vi "Autocomplete UI.vi"(0 "Allow Undefined Values? (F)":bool, 4 "LstBox Refnum":refnum<vi>, 5 "Ready Notifier":refnum<notifier>, 6 "Height (200)":i16=200, 7 "Stop Event":refnum<user-event>, 8 "Options":refnum<user-event>, 9 "Selection Event":refnum<user-event>, 10 "Autohide ListBox (F)":bool, 11 "Str Refnum":refnum<vi>) -> ()   [LabVIEW 2020, in "AutoComplete.lvlib"]
uses:
  AutoComplete.lvlib
  <vilib>/event_ctls.llb/eventvkey.ctl
panel:
  out "Revert":bool
  out "Starting Value":string
  in  "Visible":bool
  out "All Options":string[](array[string])
  in  "Listbox":i32(listbox)
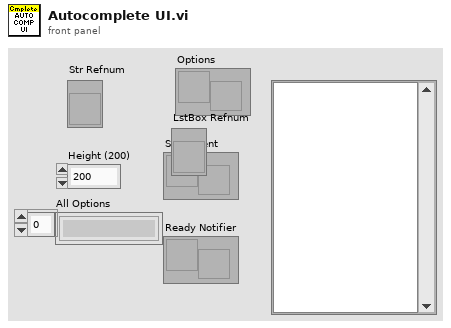
[diagram p1: front panel]
types:
  T1 = enum32{"Invalid", "Standard", "Closed", "Hidden", "Minimized", "Maximized"}
  T2 = typedef "eventvkey.ctl" = enum16{"ASCII", "Enter", "Return", "Shift", "Ctrl", "Alt", "Cmd", "Opt", "Caps", "NumLock", "Clear", "Break", "Up", "Down", "Left", "Right", "Insert", "Delete", "Home", "End", "PageUp", "PageDown", "Escape", "Help", "Pause", "ScrollLock", "F1", "F2", "F3", "F4", "F5", "F6", "F7", "F8", "F9", "F10", "F11", "F12", "F13", "F14", "F15", "F16", "F17", "F18", "F19", "F20", "F21", "F22", "F23", "F24", "Play", "VolumeUp", "VolumeDown", "Mute", "Two Byte Char"}
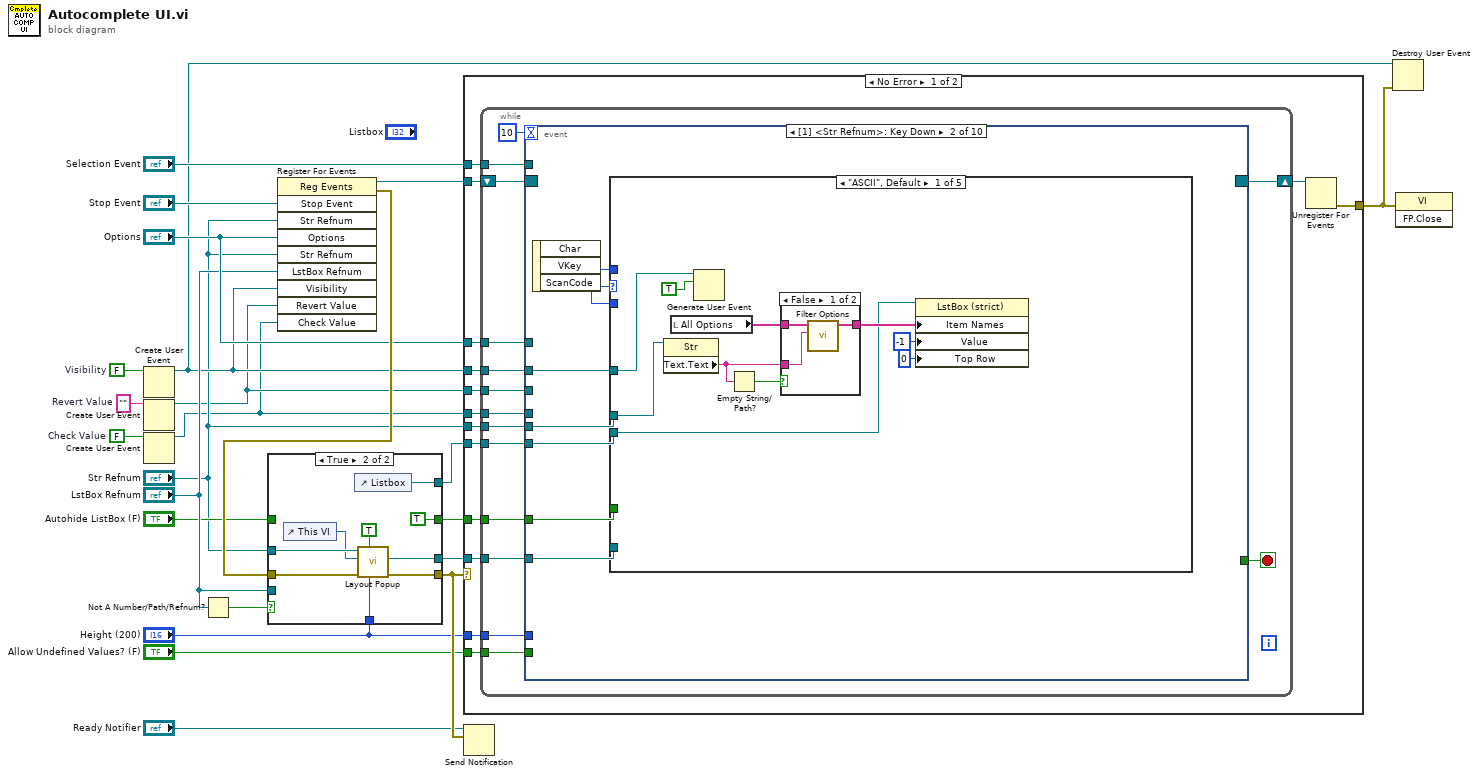
[diagram p0: block diagram]
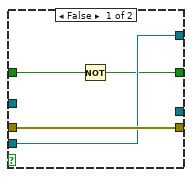
[diagram p2: hidden frame]
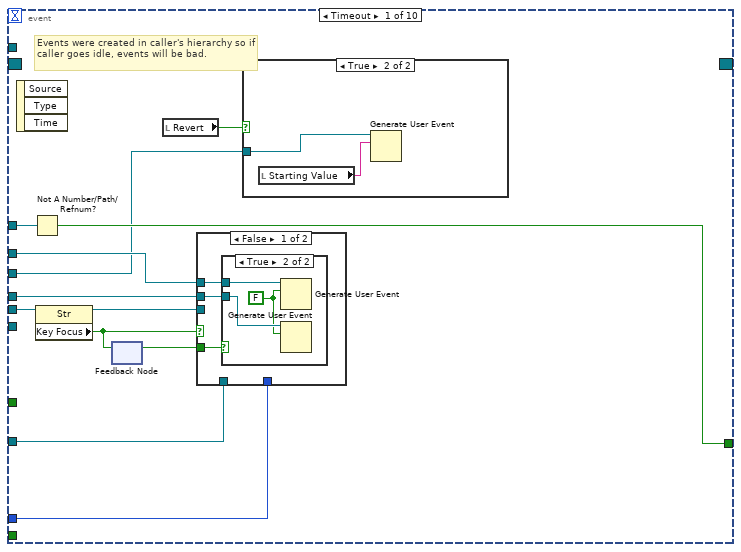
[diagram p3: hidden frame]
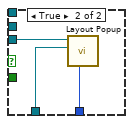
[diagram p6: hidden frame]
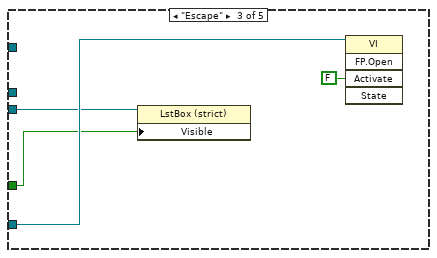
[diagram p9: hidden frame]
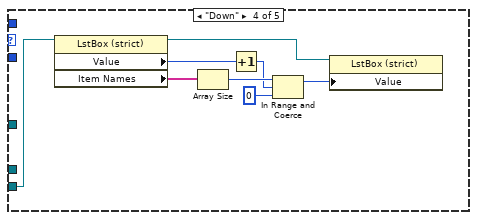
[diagram p10: hidden frame]
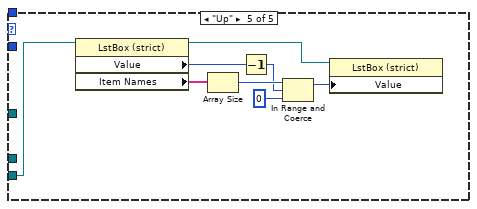
[diagram p11: hidden frame]
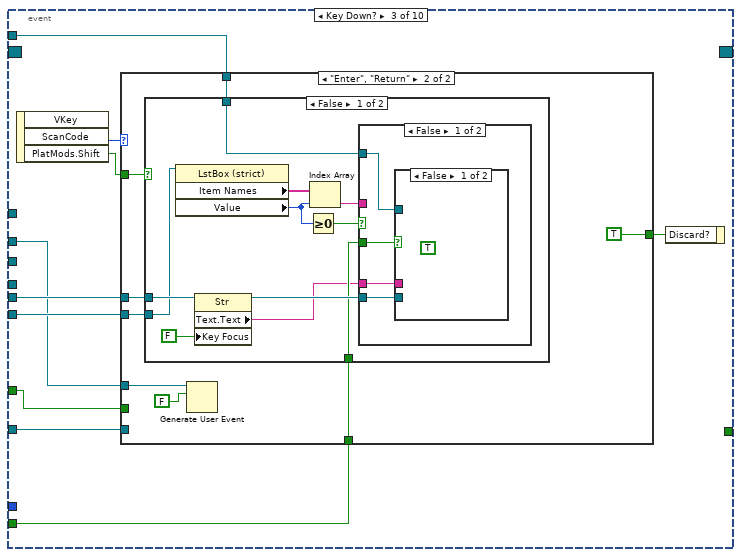
[diagram p12: hidden frame]
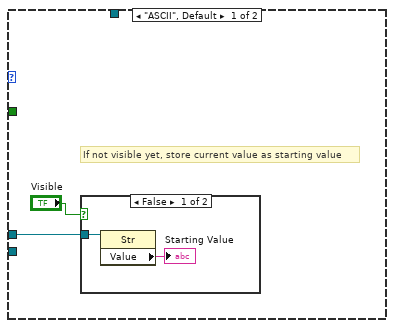
[diagram p13: hidden frame]
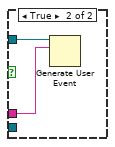
[diagram p15: hidden frame]
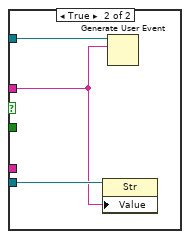
[diagram p16: hidden frame]
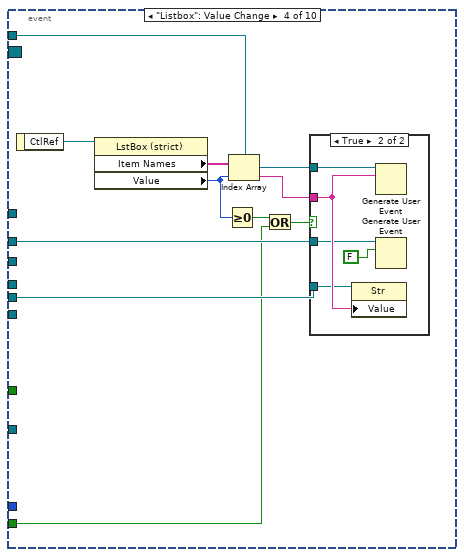
[diagram p18: hidden frame]
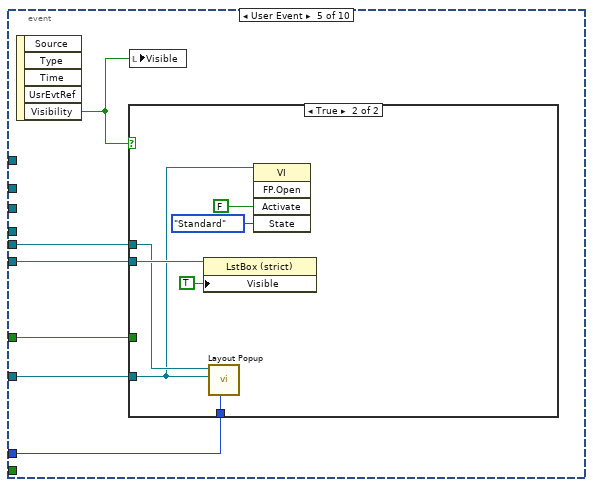
[diagram p20: hidden frame]
diagram:
  w2 = FALSE  # Check Value
  w4 = ""  # Revert Value
  w10 = FALSE  # Visibility
  n1 = Create User Event(user event datatype=w10) -> (user event=w8:refnum<user-event>)  [unwired: 1 in, 1 out]
  n2 = Create User Event(user event datatype=w4) -> (user event=w3:refnum<user-event>)  [unwired: 1 in, 1 out]
  n3 = Create User Event(user event datatype=w2) -> (user event=w1:refnum<user-event>)  [unwired: 1 in, 1 out]
  n4 = Not A Number/Path/Refnum?(number/path/refnum="LstBox Refnum") -> (NaN/Path/Refnum?=w16:bool)
  n5 = register-events("Stop Event", "Str Refnum", "Options", "Str Refnum", "LstBox Refnum", w8, w3, w1) -> (reference out=w21:refnum<event-registration>, error out=w22:errorcluster)  [unwired: 2 in]
  n6 = case shown="True" w16 {
    tunnel: w22 -> [w27 w30]
    tunnel: "Height (200)" -> [_ w32]
    tunnel: [_ w29] -> w20
    tunnel: [w27 w36] -> w23
    tunnel: "Str Refnum" -> [_ w33]
    tunnel: "LstBox Refnum" -> [w26 _]
    tunnel: [w26 w35] -> w15
    tunnel: [w24 TRUE] -> w14
    tunnel: "Autohide ListBox (F)" -> [w25 _]
    frame False {
      n7 = Not(x=w25) -> (.not. x?=w24:bool)
    }
    frame True {
      n8 = control-ref of="This VI"() -> (w31:refnum<vi>)
      n9 = control-ref of="Listbox"() -> (w35:refnum<vi>)
      n10 = call "Layout Popup.vi"("Height (200)"=w32, "Initial? (F)"=TRUE, "error in (no error)"=w30, "Popup VI In"=w31, "String Control In"=w33) -> ("error out"=w36:errorcluster, "Popup VI"=w29:refnum<vi>)  [unwired: 4 in, 1 out]
    }
  }
  n11 = case shown="No Error" w23 {
    tunnel: w21 -> [w50 _]
    tunnel: "Str Refnum" -> [w49 _]
    tunnel: [w47 _] -> w9
    tunnel: w20 -> [w46 _]
    tunnel: "Options" -> [w45 _]
    tunnel: w15 -> [w44 _]
    tunnel: w14 -> [w43 _]
    tunnel: "Selection Event" -> [w42 _]
    tunnel: w8 -> [w41 _]
    tunnel: "Height (200)" -> [w40 _]
    tunnel: "Allow Undefined Values? (F)" -> [w39 _]
    tunnel: w3 -> [w38 _]
    tunnel: w1 -> [w37 _]
    frame No Error {
      n12 = while {
        shift-right: [w64] -> w48
        shift-left: w50 -> [w65]
        tunnel: w49 -> [w62]
        tunnel: w46 -> [w60]
        tunnel: w45 -> [w59]
        tunnel: w44 -> [w58]
        tunnel: w43 -> [w57]
        tunnel: w42 -> [w56]
        tunnel: w41 -> [w55]
        tunnel: w40 -> [w54]
        tunnel: w39 -> [w53]
        tunnel: w38 -> [w52]
        tunnel: w37 -> [w51]
        stop <- w63 stop-if-true
        n13 = event shown="[1] <Str Refnum>: Key Down" {
          selector: w65 -> [_ _ _ _ _ _ _ _ _ _]
          dyn-events: [_ _ _ _ _ _ _ _ _ _] -> w64
          timeout: 10 -> [_ _ _ _ _ _ _ _ _ _]
          tunnel: [w75 _ _ _ _ TRUE _ _ _ _] -> w63
          tunnel: w62 -> [w77 w95 w137 w178 w190 _ w217 w221 w232 _]
          tunnel: w60 -> [w71 w92 w136 _ w193 _ _ _ _ _]
          tunnel: w59 -> [w76 _ _ _ _ w208 _ _ _ _]
          tunnel: w58 -> [_ w91 w135 _ w192 w211 w216 _ w231 _]
          tunnel: w57 -> [_ w90 w134 _ w191 w210 _ _ _ _]
          tunnel: w56 -> [_ _ w133 w177 _ w207 _ _ w230 _]
          tunnel: w55 -> [w74 w89 w132 w175 _ w209 _ _ _ _]
          tunnel: w54 -> [w70 _ _ _ w189 _ _ _ _ _]
          tunnel: w53 -> [_ _ w131 w173 _ _ _ _ w229 _]
          tunnel: w52 -> [w69 _ _ _ _ w206 _ _ _ _]
          tunnel: w51 -> [w66 _ _ _ _ _ _ _ _ _]
          event Timeout {
            # "Events were created in caller's hierarchy so if caller goes idle, events will be bad."
            n14 = event-data() -> ()  [unwired: 1 in, 3 out]
            n15 = Not A Number/Path/Refnum?(number/path/refnum=w76) -> (NaN/Path/Refnum?=w75:bool)
            n16 = property class="Str"(reference=w77) -> (reference out=w67:refnum<vi>, "Key Focus"=w73:bool)  [unwired: 1 in, 1 out]
            n17 = feedback-in #1(w73) -> ()
            n18 = feedback #1() -> (w72:bool)  [unwired: 1 in]
            n19 = local read "Revert"() -> (w68:bool)
            n20 = case shown="False" w73 {
              tunnel: w74 -> [w82 _]
              tunnel: w72 -> [w81 _]
              tunnel: w67 -> [_ w88]
              tunnel: w71 -> [_ w87]
              tunnel: w70 -> [_ w86]
              tunnel: w66 -> [w80 _]
              frame False {
                n21 = case shown="True" w81 {
                  tunnel: w82 -> [_ w85]
                  tunnel: w80 -> [_ w84]
                  frame False {
                  }
                  frame True {
                    w83 = FALSE ("event data")
                    n22 = Generate User Event(user event=w85, event data cluster=w83) -> ()  [unwired: 2 in, 2 out]
                    n23 = Generate User Event(user event=w84, event data cluster=w83) -> ()  [unwired: 2 in, 2 out]
                  }
                }
              }
              frame True {
                n24 = call "Layout Popup.vi"("Height (200)"=w86, "Popup VI In"=w87, "String Control In"=w88) -> ()  [unwired: 6 in, 3 out]
              }
            }
            n25 = case shown="True" w68 {
              tunnel: w69 -> [_ w79]
              frame False {
              }
              frame True {
                n26 = local read "Starting Value"() -> (w78:string)
                n27 = Generate User Event(user event=w79, event data cluster=w78) -> ()  [unwired: 2 in, 2 out]
              }
            }
          }
          event Key Down {
            n28 = event-data() -> ("Char"=w94:i16, "VKey"=w96:T2, "ScanCode"=w93:i16)  [unwired: 1 in]
            n29 = case shown="\"ASCII\", Default" w96 {
              tunnel: w95 -> [w105 _ _ _ _]
              tunnel: w94 -> [_ _ _ _ _]
              tunnel: w93 -> [_ _ _ _ _]
              tunnel: w92 -> [_ _ w113 _ _]
              tunnel: w91 -> [w99 _ w112 w116 w123]
              tunnel: w90 -> [_ _ w111 _ _]
              tunnel: w89 -> [w98 _ _ _ _]
              frame "ASCII", Default {
                n30 = property class="Str"(reference=w105) -> ("Text.Text"=w101:string)  [unwired: 1 in, 2 out]
                n31 = local read "All Options"() -> (w102:string[])
                n32 = Generate User Event(user event=w98, event data cluster=TRUE ("event data")) -> ()  [unwired: 2 in, 2 out]
                n33 = Empty String/Path?(string/path=w101) -> (empty?=w100:bool)
                n34 = case shown="False" w100 {
                  tunnel: [w107 w110] -> w103
                  tunnel: w102 -> [w109 w110]
                  tunnel: w101 -> [w108 _]
                  frame False {
                    n35 = call "Filter Options.vi"("Text"=w108, "All Options"=w109) -> ("Filtered Names"=w107:string[])  [unwired: 9 in]
                  }
                  frame True {
                  }
                }
                n36 = property on="Property Node" class="LstBox (strict)"(reference=w99, "Item Names"=w103, "Value"=-1 ("Listbox"), "Top Row"=0) -> ()  [unwired: 1 in, 2 out]
              }
              frame "Enter", "Return" {
                # "Handled in Key Down?"
              }
              frame "Escape" {
                n37 = property class="LstBox (strict)"(reference=w112, "Visible"=w111) -> ()  [unwired: 1 in, 2 out]
                n38 = invoke class="VI" method="FP.Open"(reference=w113, "Activate"=FALSE ("Activate?")) -> ()  [unwired: 3 in, 5 out]
              }
              frame "Down" {
                n39 = property on="Property Node" class="LstBox (strict)"(reference=w116) -> (reference out=w115:refnum<vi>, "Value"=w121:i32, "Item Names"=w122:string[])  [unwired: 1 in, 1 out]
                n40 = Array Size(array=w122) -> (size(s)=w120:i32)
                n41 = Increment(x=w121) -> (x+1=w119:i32)
                n42 = In Range and Coerce(upper limit=w120, x=w119, lower limit=0) -> (coerced(x)=w117:i32)  [unwired: 1 out]
                n43 = property on="Property Node" class="LstBox (strict)"(reference=w115, "Value"=w117) -> ()  [unwired: 1 in, 2 out]
              }
              frame "Up" {
                n44 = property on="Property Node" class="LstBox (strict)"(reference=w123) -> (reference out=w124:refnum<vi>, "Value"=w129:i32, "Item Names"=w130:string[])  [unwired: 1 in, 1 out]
                n45 = Array Size(array=w130) -> (size(s)=w128:i32)
                n46 = Decrement(x=w129) -> (x-1=w127:i32)
                n47 = In Range and Coerce(upper limit=w128, x=w127, lower limit=0) -> (coerced(x)=w125:i32)  [unwired: 1 out]
                n48 = property on="Property Node" class="LstBox (strict)"(reference=w124, "Value"=w125) -> ()  [unwired: 1 in, 2 out]
              }
            }
          }
          event Key Down? {
            n49 = event-data() -> ("VKey"=w140:T2, "PlatMods.Shift"=w139:bool)  [unwired: 1 in, 1 out]
            n50 = case shown="\"Enter\", \"Return\"" w140 {
              tunnel: w139 -> [_ w152]
              tunnel: [_ TRUE] -> w138
              tunnel: w137 -> [w142 w150]
              tunnel: w136 -> [_ _]
              tunnel: w135 -> [_ w149]
              tunnel: w134 -> [_ _]
              tunnel: w133 -> [_ w148]
              tunnel: w132 -> [_ w147]
              tunnel: w131 -> [_ w145]
              frame "ASCII", Default {
                # "If not visible yet, store current value as starting value"
                n51 = case shown="False" "Visible" {
                  tunnel: w142 -> [w144 _]
                  frame False {
                    n52 = property class="Str"(reference=w144) -> ("Value"=→"Starting Value":string)  [unwired: 1 in, 2 out]
                  }
                  frame True {
                  }
                }
              }
              frame "Enter", "Return" {
                n53 = case shown="False" w152 {
                  tunnel: w150 -> [w159 _]
                  tunnel: w149 -> [w157 _]
                  tunnel: w148 -> [w156 _]
                  tunnel: w145 -> [w154 _]
                  frame False {
                    n54 = property on="Property Node" class="LstBox (strict)"(reference=w157) -> ("Item Names"=w163:string[], "Value"=w162:i32)  [unwired: 1 in, 2 out]
                    n55 = property class="Str"(reference=w159, "Key Focus"=FALSE) -> (reference out=w158:refnum<vi>, "Text.Text"=w153:string)  [unwired: 1 in, 1 out]
                    n56 = Greater Or Equal To 0?(x=w162) -> (x >= 0?=w155:bool)
                    n57 = Index Array(array=w163, index=w162) -> (element=w161:string)
                    n58 = case shown="False" w155 {
                      tunnel: w161 -> [_ w170]
                      tunnel: w158 -> [w164 w172]
                      tunnel: w156 -> [w165 w171]
                      tunnel: w154 -> [w166 _]
                      tunnel: w153 -> [w167 _]
                      frame False {
                        n59 = case shown="False" w166 {
                          tunnel: w167 -> [_ w168]
                          tunnel: w165 -> [_ w169]
                          tunnel: w164 -> [_ _]
                          frame False {
                            (unwired) TRUE ("Revert")
                          }
                          frame True {
                            n60 = Generate User Event(user event=w169, event data cluster=w168) -> ()  [unwired: 2 in, 2 out]
                          }
                        }
                      }
                      frame True {
                        n61 = property class="Str"(reference=w172, "Value"=w170) -> ()  [unwired: 1 in, 2 out]
                        n62 = Generate User Event(user event=w171, event data cluster=w170) -> ()  [unwired: 2 in, 2 out]
                      }
                    }
                  }
                  frame True {
                  }
                }
                n63 = Generate User Event(user event=w147, event data cluster=FALSE ("event data")) -> ()  [unwired: 2 in, 2 out]
              }
            }
            n64 = event-data("Discard?"=w138) -> ()  [unwired: 1 in, 1 out]
          }
          event "Listbox": Value Change {
            n65 = event-data() -> ("CtlRef"=w176:refnum<vi>)  [unwired: 1 in]
            n66 = property on="Property Node" class="LstBox (strict)"(reference=w176) -> ("Item Names"=w182:string[], "Value"=w181:i32)  [unwired: 1 in, 2 out]
            n67 = Greater Or Equal To 0?(x=w181) -> (x >= 0?=w180:bool)
            n68 = Index Array(array=w182, index=w181) -> (element=w179:string)
            n69 = Or(x=w180, y=w173) -> (x .or. y?=w174:bool)
            n70 = case shown="True" w174 {
              tunnel: w179 -> [_ w187]
              tunnel: w178 -> [_ w186]
              tunnel: w177 -> [_ w185]
              tunnel: w175 -> [_ w184]
              frame False {
              }
              frame True {
                n71 = property class="Str"(reference=w186, "Value"=w187) -> ()  [unwired: 1 in, 2 out]
                n72 = Generate User Event(user event=w185, event data cluster=w187) -> ()  [unwired: 2 in, 2 out]
                n73 = Generate User Event(user event=w184, event data cluster=FALSE ("event data")) -> ()  [unwired: 2 in, 2 out]
              }
            }
          }
          event User Event {
            n74 = event-data() -> ("Visibility"=w188:bool)  [unwired: 1 in, 4 out]
            n75 = case shown="True" w188 {
              tunnel: w193 -> [w195 w200]
              tunnel: w192 -> [w197 w204]
              tunnel: w191 -> [w194 _]
              tunnel: w190 -> [_ w201]
              tunnel: w189 -> [_ w202]
              frame False {
                (unwired) FALSE
                n76 = property class="LstBox (strict)"(reference=w197, "Visible"=w194) -> ()  [unwired: 1 in, 2 out]
                n77 = invoke class="VI" method="FP.Open"(reference=w195, "Activate"=FALSE ("Activate?"), "State"=T1."Hidden") -> ()  [unwired: 2 in, 5 out]
              }
              frame True {
                n78 = property class="LstBox (strict)"(reference=w204, "Visible"=TRUE) -> ()  [unwired: 1 in, 2 out]
                n79 = call "Layout Popup.vi"("Height (200)"=w202, "Popup VI In"=w200, "String Control In"=w201) -> ()  [unwired: 6 in, 3 out]
                n80 = invoke class="VI" method="FP.Open"(reference=w200, "Activate"=FALSE ("Activate?"), "State"=T1."Standard") -> ()  [unwired: 2 in, 5 out]
              }
            }
            n81 = local write "Visible"(w188) -> ()
          }
          event User Event {
            n82 = event-data() -> ()  [unwired: 1 in, 1 out]
            n83 = Destroy User Event(user event=w207) -> ()  [unwired: 1 in, 1 out]
            n84 = Destroy User Event(user event=w206) -> ()  [unwired: 1 in, 1 out]
            n85 = Destroy User Event(user event=w209) -> ()  [unwired: 1 in, 1 out]
            n86 = property class="LstBox (strict)"(reference=w211, "Visible"=w210) -> ()  [unwired: 1 in, 2 out]
            n87 = Destroy User Event(user event=w208) -> ()  [unwired: 1 in, 1 out]
          }
          event User Event {
            # "Use this hidden indicator to store the full list of options since we'll be filtering down the displayed listbox."
            n88 = event-data() -> ("Options"=w215:string[])  [unwired: 1 in]
            "All Options" <- w215
            n89 = property class="Str"(reference=w217) -> ("Text.Text"=w214:string)  [unwired: 1 in, 2 out]
            n90 = call "Filter Options.vi"("Text"=w214, "All Options"=w215) -> ("Filtered Names"=w213:string[])  [unwired: 9 in]
            n91 = property on="Property Node" class="LstBox (strict)"(reference=w216, "Item Names"=w213, "Value"=-1 ("Listbox"), "Top Row"=0) -> ()  [unwired: 1 in, 2 out]
          }
          event User Event {
            n92 = event-data() -> ("Revert Value"=w220:string)  [unwired: 1 in]
            n93 = property class="Str"(reference=w221, "Value"=w220) -> ()  [unwired: 1 in, 2 out]
            n94 = call <vilib>:"Beep.vi"() -> ()  [unwired: 12 in]
          }
          event User Event {
            n95 = event-data() -> ()  [unwired: 1 in, 1 out]
            n96 = property on="Property Node" class="LstBox (strict)"(reference=w231) -> ("Item Names"=w222:string[], "Value"=w228:i32)  [unwired: 1 in, 2 out]
            n97 = property class="Str"(reference=w232, "Key Focus"=FALSE) -> (reference out=w225:refnum<vi>, "Text.Text"=w223:string)  [unwired: 1 in, 1 out]
            n98 = Index Array(array=w222, index=w228) -> (element=w227:string)
            n99 = Greater Or Equal To 0?(x=w228) -> (x >= 0?=w224:bool)
            n100 = case shown="False" w224 {
              tunnel: w227 -> [_ w248]
              tunnel: w225 -> [w234 w250]
              tunnel: w230 -> [w235 w249]
              tunnel: w229 -> [w236 _]
              tunnel: w223 -> [w237 _]
              tunnel: w222 -> [w233 _]
              frame False {
                n101 = case shown="False" w236 {
                  tunnel: w237 -> [w238 w246]
                  tunnel: w235 -> [w239 w247]
                  tunnel: w234 -> [_ _]
                  tunnel: w233 -> [w242 _]
                  frame False {
                    n102 = Search 1D Array(1D array=w242, element=w238) -> (index of element=w241:i32)  [unwired: 1 in]
                    n103 = Less Than 0?(x=w241) -> (x < 0?=w240:bool)
                    n104 = case shown="True" w240 {
                      tunnel: w239 -> [w244 _]
                      tunnel: w238 -> [w243 _]
                      frame False {
                        n105 = Generate User Event(user event=w244, event data cluster=w243) -> ()  [unwired: 2 in, 2 out]
                      }
                      frame True {
                        "Revert" <- TRUE ("Revert")
                      }
                    }
                  }
                  frame True {
                    n106 = Generate User Event(user event=w247, event data cluster=w246) -> ()  [unwired: 2 in, 2 out]
                  }
                }
              }
              frame True {
                n107 = property class="Str"(reference=w250, "Value"=w248) -> ()  [unwired: 1 in, 2 out]
                n108 = Generate User Event(user event=w249, event data cluster=w248) -> ()  [unwired: 2 in, 2 out]
              }
            }
          }
          event Key Down {
            n109 = event-data() -> ("VKey"=w252:T2)  [unwired: 1 in]
            n110 = Equal?(x=w252, y=eventvkey."Escape") -> ()  [unwired: 1 out]
          }
        }
      }
      n111 = Unregister For Events(event registration refnum=w48) -> (error out=w47:errorcluster)  [unwired: 1 in]
    }
    frame Error {
    }
  }
  n112 = Send Notification(notification=w23, notifier="Ready Notifier") -> ()  [unwired: 1 in, 2 out]
  n113 = Destroy User Event(user event=w8, error in=w9) -> ()  [unwired: 1 out]
  n114 = invoke class="VI" method="FP.Close"(error in=w9) -> ()  [unwired: 2 in, 3 out]
